vi "Force Channel.vi"(6 "Force Data":u8[](array[numeric]) format="%.0x", 8 "error in (no error)":errorcluster, 9 "Force Active":bool, 10 "Subscriber Name":string, 11 "CIFChannelMng in":refnum<class "CIFChannelMng.lvclass">) -> (0 "error out":errorcluster, 3 "CIFChannelMng out":refnum<class "CIFChannelMng.lvclass">)   [LabVIEW 2021, in "CIFChannelMng.lvclass"]
uses:
  CIFChannelMng.lvclass
  CIFChannelMng.lvclass/CIFChannelMng.ctl
  CIFChannels/CIFChannels.lvclass/CIFChannels.ctl
  CIFChannels/Accessors/Read Forced.vi
  ChannelCommon/Utilities/Add Error.vi
  <vilib>/CIF Foundation/CIF Utilities/Errors/Append Error Location.vi
  CIFChannels/CIFChannels.lvclass
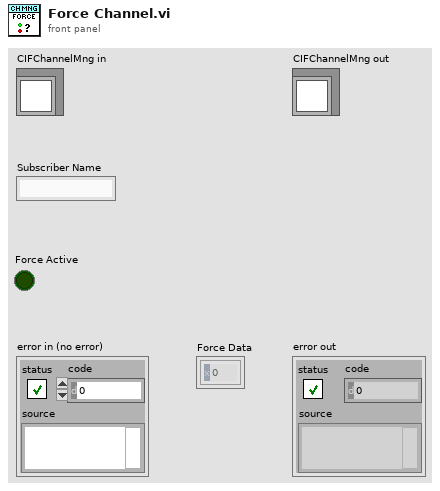
[diagram p1: front panel]
types:
  T1 = typedef "CIFChannelMng.lvclass/Channel List for OOB.ctl" = cluster{"Name":string, "Direction":T2, "Type":string, "Connected?":bool, "Connected Name":string, "Custom Config Data":u8[], "Forced?":bool}
  T2 = typedef "CIFChannels.lvclass/Direction.ctl" = enum16{"Publisher", "Subscriber"}
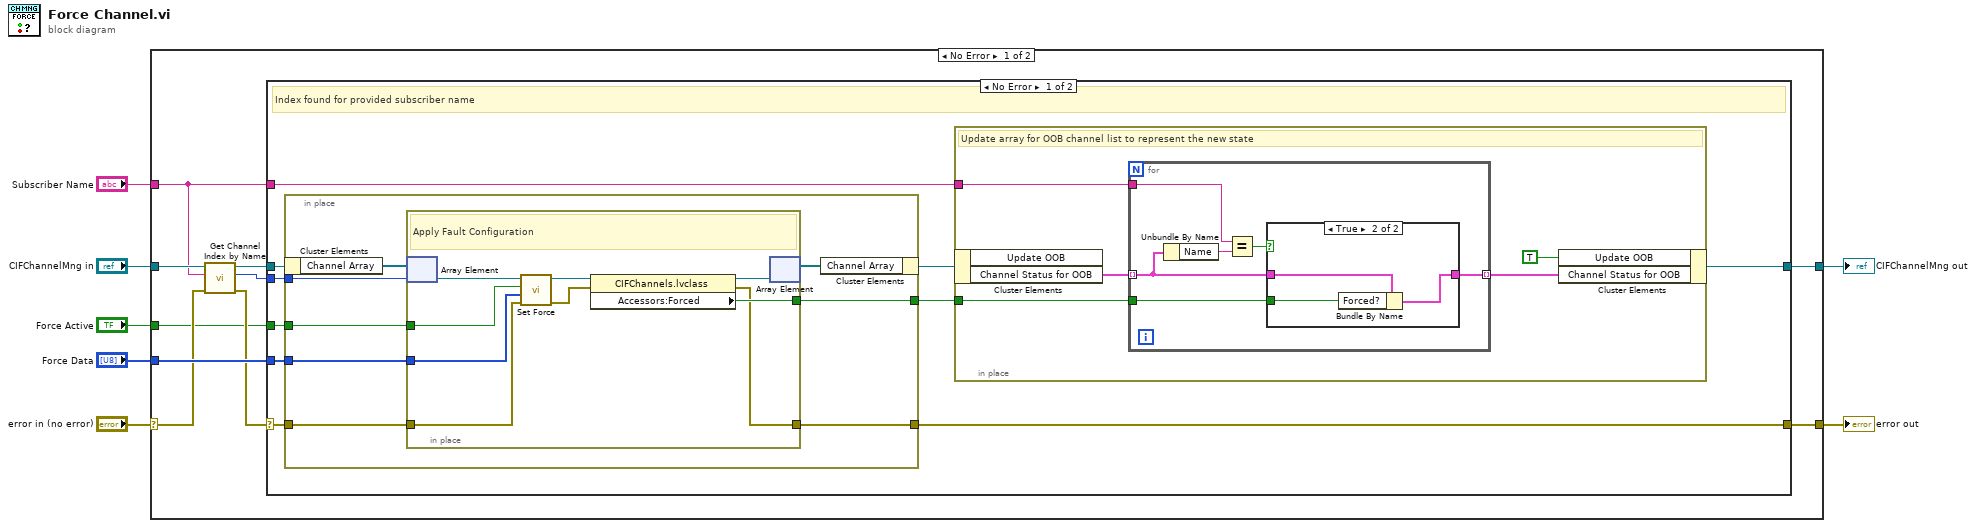
[diagram p0: block diagram]
diagram:
  n1 = case shown="No Error" "error in (no error)" {
    selector: "error in (no error)" -> [w15 w62]
    tunnel: [w10 w63] -> w5
    tunnel: "CIFChannelMng in" -> [w16 w63]
    tunnel: "Subscriber Name" -> [w11 _]
    tunnel: "Force Data" -> [w17 _]
    tunnel: [w9 w62] -> w2
    tunnel: "Force Active" -> [w8 _]
    frame No Error {
      n2 = call "Get Channel Index by Name.vi"("error in (no error)"=w15, "Channel Name"=w11, "CIFChannelMng in"=w16) -> ("error out"=w12:errorcluster, "Channel Index"=w13:i32, "CIFChannelMng out"=w14:refnum<class "CIFChannelMng.lvclass">)  [unwired: 6 in]
      n3 = case shown="No Error" w12 {
        selector: w12 -> [w24 w61]
        tunnel: w17 -> [w27 _]
        tunnel: w14 -> [w26 w60]
        tunnel: w13 -> [w25 _]
        tunnel: w11 -> [w21 _]
        tunnel: [w20 w60] -> w10
        tunnel: [w19 w61] -> w9
        tunnel: w8 -> [w18 _]
        frame No Error {
          # "Index found for provided subscriber name"
          n4 = in-place {
            in-place-border: w27 -> [w50]
            in-place-border: [w49] -> w22
            in-place-border: w25 -> [w47]
            in-place-border: w24 -> [w46]
            in-place-border: [w44] -> w19
            in-place-border: w18 -> [w43]
            n5 = in-place-cluster #1(w26) -> ("Channel Array"=w48:refnum<class "CIFChannels.lvclass">[])
            n6 = in-place {
              in-place-border: w50 -> [w59]
              in-place-border: [w52] -> w49
              in-place-border: w46 -> [w57]
              in-place-border: [w51] -> w44
              in-place-border: w43 -> [w56]
              # "Apply Fault Configuration"
              n7 = in-place-array #2(w48, w47) -> (w58:refnum<class "CIFChannels.lvclass">)
              n8 = call "Set Force.vi"("error in (no error)"=w57, "Force Data"=w59, "Force Active"=w56, "CIFChannels in"=w58) -> ("error out"=w53:errorcluster, "CIFChannels out"=w55:refnum<class "CIFChannels.lvclass">)  [unwired: 6 in]
              n9 = property class="CIFChannels.lvclass"(reference=w55, error in=w53) -> (reference out=w54:refnum<class "CIFChannels.lvclass">, error out=w51:errorcluster, "Accessors:Forced"=w52:bool)
              n10 = in-place-array #2(w54) -> (w45:refnum<class "CIFChannels.lvclass">[])  [unwired: 1 out]
            }
            n11 = in-place-cluster #1("Channel Array"=w45) -> (w23:refnum<class "CIFChannelMng.lvclass">)
          }
          n12 = in-place {
            in-place-border: w22 -> [w28]
            in-place-border: w21 -> [w29]
            # "Update array for OOB channel list to represent the new state"
            n13 = in-place-cluster #3(w23) -> ("Channel Status for OOB"=w32:T1[])  [unwired: 1 out]
            n14 = for {
              tunnel: w32 -> [w37] mode=indexing
              tunnel: w28 -> [w36]
              tunnel: [w35] -> w31 mode=indexing
              tunnel: w29 -> [w33]
              n15 = Unbundle By Name(w37) -> ("Name"=w38:string)
              n16 = Equal?(x=w33, y=w38) -> (x = y?=w34:bool)
              n17 = case shown="True" w34 {
                tunnel: w37 -> [w39 w42]
                tunnel: w36 -> [_ w41]
                tunnel: [w39 w40] -> w35
                frame False {
                }
                frame True {
                  n18 = Bundle By Name(cluster=w42, "Forced?"=w41) -> (w40:T1)
                }
              }
            }
            n19 = in-place-cluster #3("Update OOB"=TRUE, "Channel Status for OOB"=w31) -> (w20:refnum<class "CIFChannelMng.lvclass">)
          }
        }
        frame Error {
          # "Index by name created error"
        }
      }
    }
    frame Error {
    }
  }
  "error out" <- w2
  "CIFChannelMng out" <- w5
